vi "Rx Message to Map Key.vi"(10 "message":T2={"name"="", "message type"="BC to RT", "endpoint Rx"={"terminal address"=0, "subaddress"=0}, "endpoint Tx"={"terminal address"=0, "subaddress"=0}, "mode code"=0, "number of words"=0, "parameters"=[], "create timestamp channel"=FALSE}, 11 "HW channel":u16) -> (3 "message map key":T1)   [LabVIEW 2020, in "Ballard MIL-STD-1553 Engine.lvlib" / "Custom Device.lvlib"]
uses:
  Custom Device.lvlib
  Shared/Message Definition.ctl
  Shared/Message Type.ctl
  Shared/Terminal Endpoint.ctl
  Shared/Address.ctl
  Shared/Parameter Definition.ctl
  Shared/Message Map Key.ctl
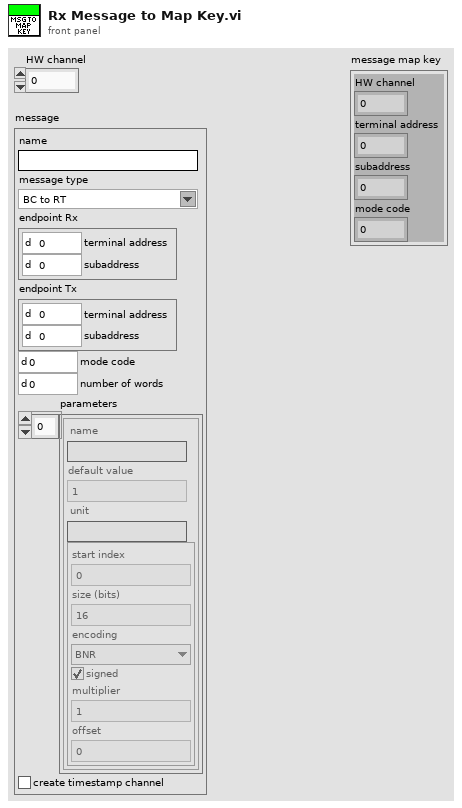
[diagram p1: front panel]
types:
  T1 = typedef "Message Map Key.ctl" = cluster{"HW channel":u16, "terminal address":u16, "subaddress":u16, "mode code":u16}
  T2 = typedef "Message Definition.ctl" = cluster{"name":string, "message type":T3, "endpoint Rx":T4, "endpoint Tx":T4, "mode code":u16, "number of words":u16, "parameters":cluster{"name":string, "default value":dbl, "unit":string, "parameter definition":T6}[], "create timestamp channel":bool}
  T3 = typedef "Message Type.ctl" = string
  T4 = typedef "Terminal Endpoint.ctl" = cluster{"terminal address":T5, "subaddress":T5}
  T5 = typedef "Address.ctl" = u16
  T6 = typedef "Parameter Definition.ctl" = cluster{"start index":i32, "size (bits)":i32, "encoding":enum16{"BNR", "BCD", "Discrete"}, "signed":bool, "multiplier":dbl, "offset":dbl}
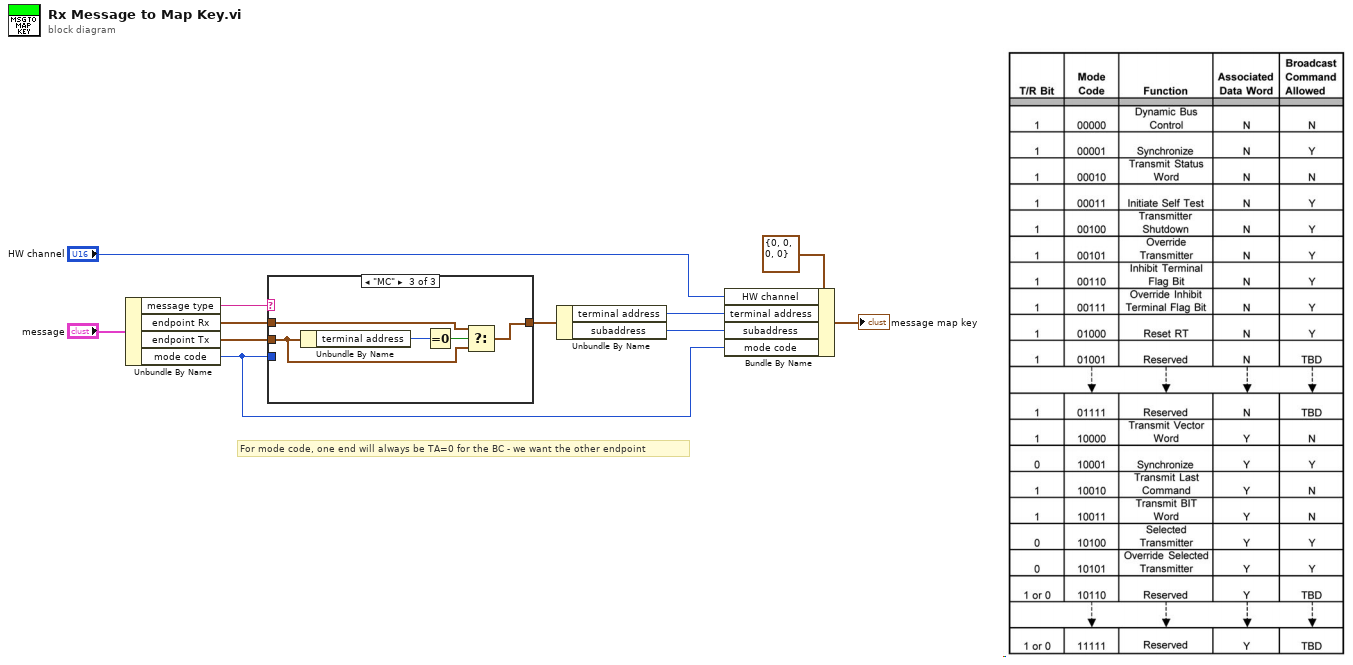
[diagram p0: block diagram]
diagram:
  # "For mode code, one end will always be TA=0 for the BC - we want the other endpoint"
  n1 = Unbundle By Name("message") -> ("message type"=w9:T3, "endpoint Rx"=w8:T4, "endpoint Tx"=w7:T4, "mode code"=w2:u16)
  n2 = case shown="\"MC\"" w9 {
    tunnel: w8 -> [w12 _ w16]
    tunnel: w7 -> [_ w13 w15]
    tunnel: w2 -> [_ _ _]
    tunnel: [w12 w13 w14] -> w3
    frame "BC to RT", "RT to RT", Default {
    }
    frame "RT to BC" {
    }
    frame "MC" {
      n3 = Unbundle By Name(w15) -> ("terminal address"=w18:T5)
      n4 = Equal To 0?(x=w18) -> (x = 0?=w17:bool)
      n5 = Select(t=w16, s=w17, f=w15) -> (s? t:f=w14:T4)
    }
  }
  n6 = Unbundle By Name(w3) -> ("terminal address"=w5:T5, "subaddress"=w4:T5)
  n7 = Bundle By Name(cluster=T1 {"HW channel"=0, "terminal address"=0, "subaddress"=0, "mode code"=0} ("message map key"), "HW channel"="HW channel", "terminal address"=w5, "subaddress"=w4, "mode code"=w2) -> (→"message map key":T1)
